vi "Theil-Sen.vi"(5 "match_lengths (T)":bool=TRUE, 6 "error in (no error)":errorcluster, 7 "Sen parameter (Auto)":enum16{"Auto", "On", "Off"}(ring), 8 "input_X":dbl[](array[numeric]), 9 "input_Y":dbl[](array[numeric])) -> (0 "error out":errorcluster, 1 "b":dbl format="%.6g", 2 "m":dbl format="%.6g", 3 "output_Y":dbl[](array[numeric]))   [LabVIEW 2021]
doc: "The Theil–Sen estimator of a set of two-dimensional points (xi, yi) is the median m of the slopes (yj - yi)/(xj - xi) determined by all pairs of sample points. Sen extended this definition to handle the case in which two data points have the same x coordinate. In Sen's definition, one takes the median of the slopes defined only from pairs of points having distinct x coordinates.\nOnce the slope m has been determined, one may determine a line from the sample points by setting the y-intercept b to be the median of the values yi - mxi. The fit line is then the line y = mx + b with coefficients m and b in slope–intercept form."
uses:
  <vilib>/Analysis/NI_AALBase.lvlib
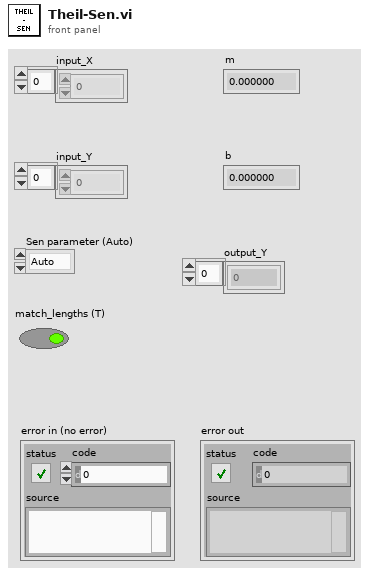
[diagram p1: front panel]
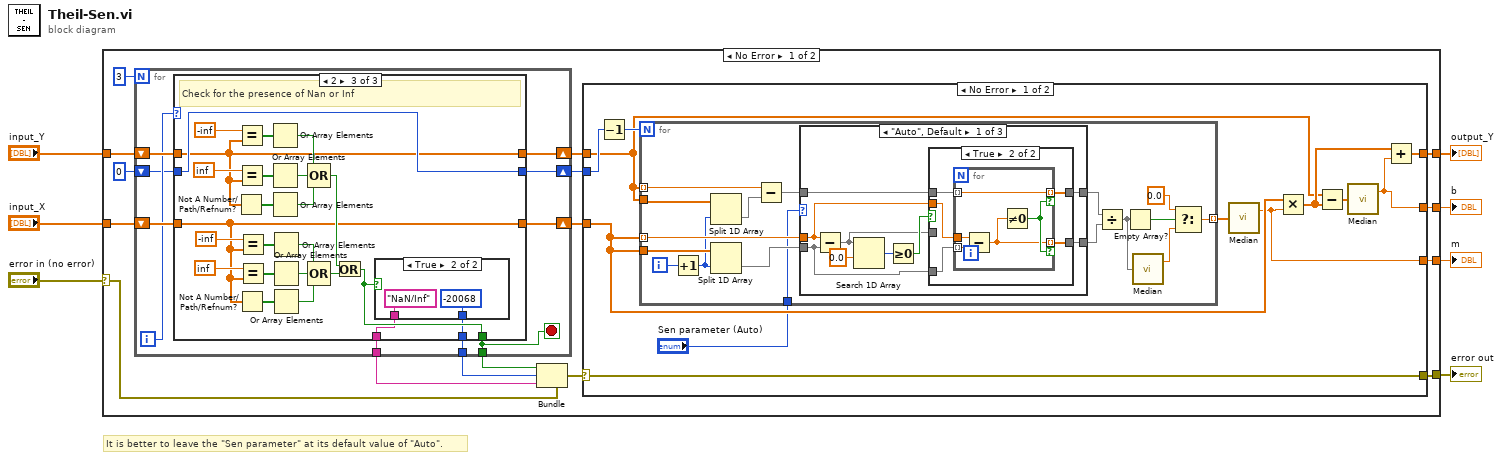
[diagram p0: block diagram]
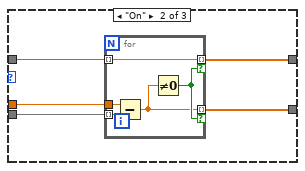
[diagram p3: hidden frame]
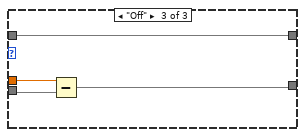
[diagram p4: hidden frame]
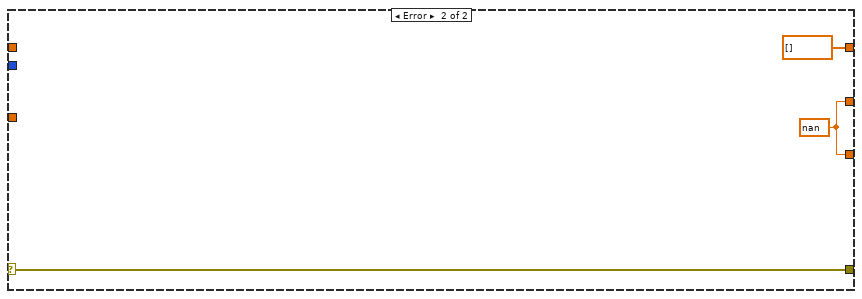
[diagram p5: hidden frame]
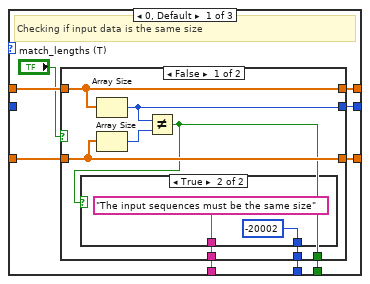
[diagram p6: hidden frame]
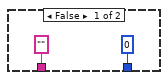
[diagram p7: hidden frame]
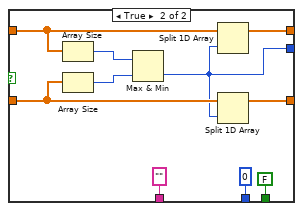
[diagram p8: hidden frame]
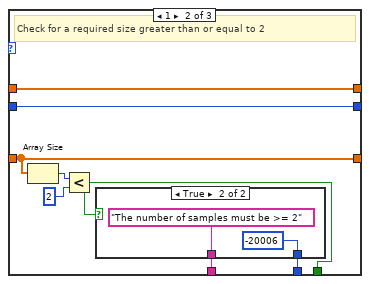
[diagram p9: hidden frame]
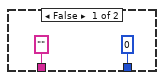
[diagram p10: hidden frame]
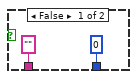
[diagram p11: hidden frame]
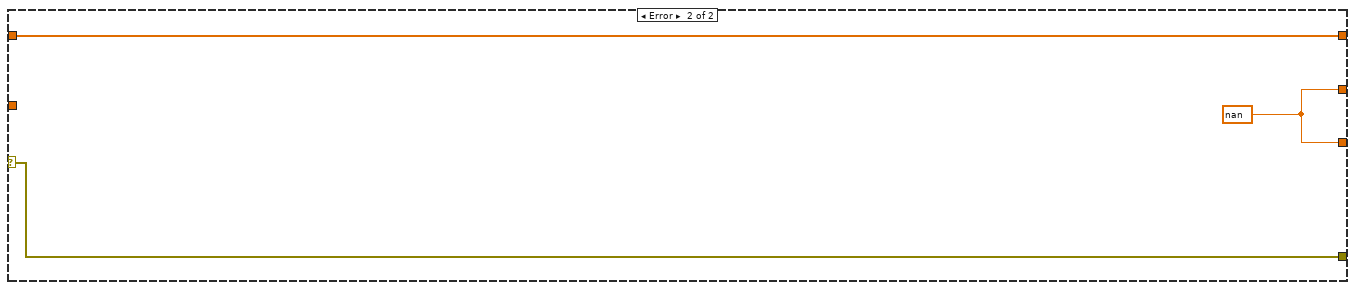
[diagram p12: hidden frame]
diagram:
  # "It is better to leave the \"Sen parameter\" at its default value of \"Auto\"."
  n1 = case shown="No Error" "error in (no error)" {
    selector: "error in (no error)" -> [w17 w173]
    tunnel: "input_X" -> [w23 _]
    tunnel: "input_Y" -> [w21 w172]
    tunnel: [w9 w173] -> w5
    tunnel: [w16 w172] -> w3
    tunnel: [w13 w171] -> w2
    tunnel: [w12 w171] -> w1
    frame No Error {
      n2 = for {
        N: 3 -> [_]
        tunnel: [w92] -> w20
        tunnel: [w97] -> w19
        tunnel: [w96] -> w18
        shift-right: [w94] -> w14
        shift-left: w21 -> [w98]
        shift-right: [w99] -> w22
        shift-left: w23 -> [w100]
        shift-right: [w95] -> w15
        shift-left: 0 -> [w91]
        i -> [w93]
        stop <- w92 stop-if-true
        n3 = case shown="2" w93 {
          tunnel: w100 -> [w109 w136 w144]
          tunnel: [w108 w136 w144] -> w99
          tunnel: w98 -> [w107 w137 w145]
          tunnel: [w105 w131 w147] -> w92
          tunnel: [w104 w132 w146] -> w97
          tunnel: [w103 w133 w143] -> w96
          tunnel: [w102 w138 w148] -> w95
          tunnel: [w101 w137 w145] -> w94
          tunnel: w91 -> [_ w138 w148]
          frame 0, Default {
            # "Checking if input data is the same size"
            n4 = case shown="False" "match_lengths (T)" {
              tunnel: w109 -> [w116 w128]
              tunnel: [w116 w127] -> w108
              tunnel: w107 -> [w115 w126]
              tunnel: [w115 w125] -> w101
              tunnel: [w111 FALSE] -> w105
              tunnel: [w113 0] -> w104
              tunnel: [w112 ""] -> w103
              tunnel: [w110 w124] -> w102
              frame False {
                n5 = Array Size(array=w115) -> (size(s)=w110:i32)
                n6 = Array Size(array=w116) -> (size(s)=w114:i32)
                n7 = Not Equal?(x=w110, y=w114) -> (x != y?=w111:bool)
                n8 = case shown="True" w111 {
                  tunnel: [0 -20002] -> w113
                  tunnel: ["" "The input sequences must be the same size"] -> w112
                  frame False {
                  }
                  frame True {
                  }
                }
              }
              frame True {
                n9 = Array Size(array=w126) -> (size(s)=w130:i32)
                n10 = Array Size(array=w128) -> (size(s)=w129:i32)
                n11 = Max & Min(x=w130, y=w129) -> (min(x,y)=w124:i32)  [unwired: 1 out]
                n12 = Split 1D Array(array=w126, index=w124) -> (first subarray=w125:dbl[])  [unwired: 1 out]
                n13 = Split 1D Array(array=w128, index=w124) -> (first subarray=w127:dbl[])  [unwired: 1 out]
              }
            }
          }
          frame 1 {
            # "Check for a required size greater than or equal to 2"
            n14 = Array Size(array=w136) -> (size(s)=w135:i32)
            n15 = Less?(x=w135, y=2) -> (x < y?=w131:bool)
            n16 = case shown="True" w131 {
              tunnel: [0 -20006] -> w132
              tunnel: ["" "The number of samples must be >= 2"] -> w133
              frame False {
              }
              frame True {
              }
            }
          }
          frame 2 {
            # "Check for the presence of Nan or Inf"
            n17 = Not A Number/Path/Refnum?(number/path/refnum=w145) -> (NaN/Path/Refnum?=w166:bool[])
            n18 = Equal?(x=-inf, y=w145) -> (x = y?=w162:bool[])
            n19 = Equal?(x=inf, y=w145) -> (x = y?=w163:bool[])
            n20 = Not A Number/Path/Refnum?(number/path/refnum=w144) -> (NaN/Path/Refnum?=w151:bool[])
            n21 = Equal?(x=-inf, y=w144) -> (x = y?=w155:bool[])
            n22 = Equal?(x=inf, y=w144) -> (x = y?=w154:bool[])
            n23 = Or Array Elements(Boolean array=w162) -> (logical OR=w160:bool)
            n24 = Or Array Elements(Boolean array=w163) -> (logical OR=w161:bool)
            n25 = Or Array Elements(Boolean array=w166) -> (logical OR=w159:bool)
            n26 = Or Array Elements(Boolean array=w155) -> (logical OR=w157:bool)
            n27 = Or Array Elements(Boolean array=w154) -> (logical OR=w156:bool)
            n28 = Or Array Elements(Boolean array=w151) -> (logical OR=w158:bool)
            n29 = Compound Arithmetic op=OR(w160, w161, w159) -> (w150:bool)
            n30 = Compound Arithmetic op=OR(w157, w156, w158) -> (w149:bool)
            n31 = Or(x=w150, y=w149) -> (x .or. y?=w147:bool)
            n32 = case shown="True" w147 {
              tunnel: [0 -20068] -> w146
              tunnel: ["" "NaN/Inf"] -> w143
              frame False {
              }
              frame True {
              }
            }
          }
        }
      }
      n33 = Bundle(cluster=w17, "status"=w20, "code"=w19, "source"=w18) -> (w10:errorcluster)
      n34 = case shown="No Error" w10 {
        selector: w10 -> [w24 w90]
        tunnel: w22 -> [w35 _]
        tunnel: [w30 dbl[] []] -> w16
        tunnel: w15 -> [w29 _]
        tunnel: w14 -> [w28 _]
        tunnel: [w26 w88] -> w13
        tunnel: [w25 w88] -> w12
        tunnel: [w24 w90] -> w9
        frame No Error {
          n35 = Decrement(x=w29) -> (x-1=w34:i32)
          n36 = for {
            N: w34 -> [_]
            tunnel: w35 -> [w50] mode=indexing
            tunnel: w28 -> [w51]
            tunnel: w35 -> [w52]
            tunnel: [w38] -> w33 mode=indexing
            tunnel: w28 -> [w42] mode=indexing
            tunnel: "Sen parameter (Auto)" -> [w41]
            i -> [w47]
            n37 = Increment(x=w47) -> (x+1=w46:i32)
            n38 = Split 1D Array(array=w51, index=w46) -> (second subarray=w48:dbl[])  [unwired: 1 out]
            n39 = Split 1D Array(array=w52, index=w46) -> (second subarray=w49:dbl[])  [unwired: 1 out]
            n40 = Subtract(x=w42, y=w48) -> (x-y=w44:dbl[])
            n41 = case shown="\"Auto\", Default" w41 {
              tunnel: w50 -> [w55 w78 w86]
              tunnel: w49 -> [w54 w77 w85]
              tunnel: [w60 w76 w84] -> w45
              tunnel: w44 -> [w59 w75 w87]
              tunnel: [w61 w74 w87] -> w43
              frame "Auto", Default {
                n42 = Subtract(x=w55, y=w54) -> (x-y=w53:dbl[])
                n43 = Search 1D Array(1D array=w53, element=0.0) -> (index of element=w57:i32)  [unwired: 1 in]
                n44 = Greater Or Equal To 0?(x=w57) -> (x >= 0?=w56:bool)
                n45 = case shown="True" w56 {
                  tunnel: [w63 w68] -> w61
                  tunnel: [w62 w67] -> w60
                  tunnel: w59 -> [w63 w66]
                  tunnel: w55 -> [_ w65]
                  tunnel: w54 -> [_ w64]
                  tunnel: w53 -> [w62 _]
                  frame False {
                  }
                  frame True {
                    n46 = for {
                      tunnel: w65 -> [w73]
                      tunnel: w64 -> [w72] mode=indexing
                      tunnel: [w69] -> w67 mode=indexing if=w70
                      tunnel: [w71] -> w68 mode=indexing if=w70
                      tunnel: w66 -> [w71] mode=indexing
                      n47 = Subtract(x=w73, y=w72) -> (x-y=w69:dbl)
                      n48 = Not Equal To 0?(x=w69) -> (x != 0?=w70:bool)
                    }
                  }
                }
              }
              frame "On" {
                n49 = for {
                  tunnel: w78 -> [w83]
                  tunnel: w77 -> [w82] mode=indexing
                  tunnel: [w79] -> w76 mode=indexing if=w80
                  tunnel: [w81] -> w74 mode=indexing if=w80
                  tunnel: w75 -> [w81] mode=indexing
                  n50 = Subtract(x=w83, y=w82) -> (x-y=w79:dbl)
                  n51 = Not Equal To 0?(x=w79) -> (x != 0?=w80:bool)
                }
              }
              frame "Off" {
                n52 = Subtract(x=w86, y=w85) -> (x-y=w84:dbl[])
              }
            }
            n53 = Divide(x=w43, y=w45) -> (x/y=w39:dbl[])
            n54 = Empty Array?(array=w39) -> (empty?=w40:bool)
            n55 = call <vilib>:"Median.vi"("X"=w39) -> ("median"=w37:dbl)  [unwired: 1 out]
            n56 = Select(t=0.0, s=w40, f=w37) -> (s? t:f=w38:dbl)
          }
          n57 = call <vilib>:"Median.vi"("X"=w33) -> ("median"=w25:dbl)  [unwired: 1 out]
          n58 = Multiply(x=w35, y=w25) -> (x*y=w31:dbl[])
          n59 = Subtract(x=w28, y=w31) -> (x-y=w32:dbl[])
          n60 = call <vilib>:"Median.vi"("X"=w32) -> ("median"=w26:dbl)  [unwired: 1 out]
          n61 = Add(x=w31, y=w26) -> (x+y=w30:dbl[])
        }
        frame Error {
          w88 = nan
        }
      }
    }
    frame Error {
      w171 = nan
    }
  }
  "error out" <- w5
  "output_Y" <- w3
  "b" <- w2
  "m" <- w1
